vi "Colorize3D.vi"(8 "ColorMap":T1=52 items=["Bathymetry9", "BlackBody", "Blue", "BlueBlackRed", "BlueGreenOrange", "BlueHot", "BlueHot256", "BlueRedGreen", "BlueRedGreen256", "BrownViolet", "Classification", "ColdWarm", "Copper", "Cyan", "CyanMagenta", "Cycles", "dBZ14", "dBZ21", "EOSOrangeBlue11", "EOSSpectral11", "Fiddle", "Geo", "Geo32", "Gold", "Grays", "Grays16", "Grays256", "Green", "GreenMagenta16", "LandAndSea", "LandAndSea8", "Magenta", "Mocha", "Mud", "Pastels", "PastelsMap", "PastelsMap20", "PlanetEarth", "PlanetEarth256", "Rainbow", "Rainbow4Cycles", "Rainbow16", "Rainbow256", "RainbowCycle", "Red", "RedWhiteBlue", "RedWhiteBlue256", "RedWhiteGreen", "Relief", "Relief19", "SeaLandAndFire", "Spectrum", "SpectrumBlack", "Terrain", "Terrain256", "VioletOrangeYellow", "Web216", "Yellow", "YellowHot", "YellowHot256"], 9 "Low":dbl, 10 "High":dbl=1.0, 11 "StackIn":u16[][][](array[numeric])) -> (3 "Colorized":u32[][][](array[numeric]))   [LabVIEW 2014]
uses:
  ColorMaps.ctl
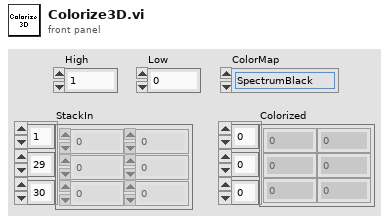
[diagram p1: front panel]
types:
  T1 = typedef "ColorMaps.ctl" = u16
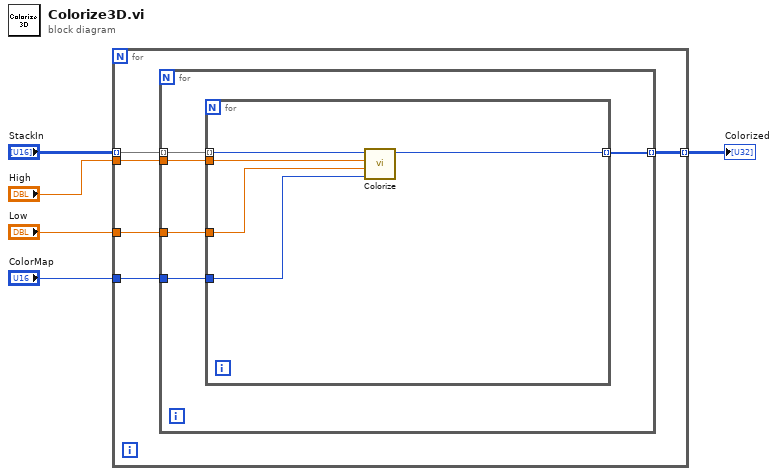
[diagram p0: block diagram]
diagram:
  n1 = for {
    tunnel: "StackIn" -> [w10] mode=indexing
    tunnel: [w9] -> w4 mode=indexing
    tunnel: "High" -> [w8]
    tunnel: "Low" -> [w7]
    tunnel: "ColorMap" -> [w6]
    n2 = for {
      tunnel: w10 -> [w15] mode=indexing
      tunnel: [w14] -> w9 mode=indexing
      tunnel: w8 -> [w13]
      tunnel: w7 -> [w12]
      tunnel: w6 -> [w11]
      n3 = for {
        tunnel: w15 -> [w20] mode=indexing
        tunnel: [w19] -> w14 mode=indexing
        tunnel: w13 -> [w18]
        tunnel: w12 -> [w17]
        tunnel: w11 -> [w16]
        n4 = call "Colorize.vi"("ColorMap"=w16, "Low"=w17, "High"=w18, "ValueIn"=w20) -> ("ColorOut"=w19:u32)  [unwired: 7 in]
      }
    }
  }
  "Colorized" <- w4
